vi "Get Indicators RegisterMap.vi"(8 "error in (no error)":errorcluster, 11 "Item Ref in":T1 format="%.0x") -> (0 "error out":errorcluster, 2 "Indicators RegisterMap":T2[](array[typedef]) {"Address" format="%.0x"}, 3 "Item Ref out":T1 format="%.0x")   [LabVIEW 2016, in "FPGA Addon System Explorer.lvlib"]
uses:
  FPGA Addon System Explorer.lvlib
  <vilib>/rvi/Bitfile/nirviControlStructure.ctl
  <vilib>/rvi/Bitfile/nirviTypdefDescription.ctl
  <vilib>/rvi/Bitfile/nirviMechanicalAction.ctl
  <vilib>/rvi/Bitfile/nirviSubControlStructure.ctl
  <vilib>/rvi/Bitfile/nirviClusterElementControl.ctl
  <vilib>/NI Veristand/Custom Device API/Custom Device Item Ref.ctl
  <vilib>/NI Veristand/Custom Device API/Get Item Property (Variant).vi
  Shared/Constants.vi
  Shared/FPGA Addon Shared.lvlib
  <vilib>/NI VeriStand/Custom Device API/Custom Device API.lvlib
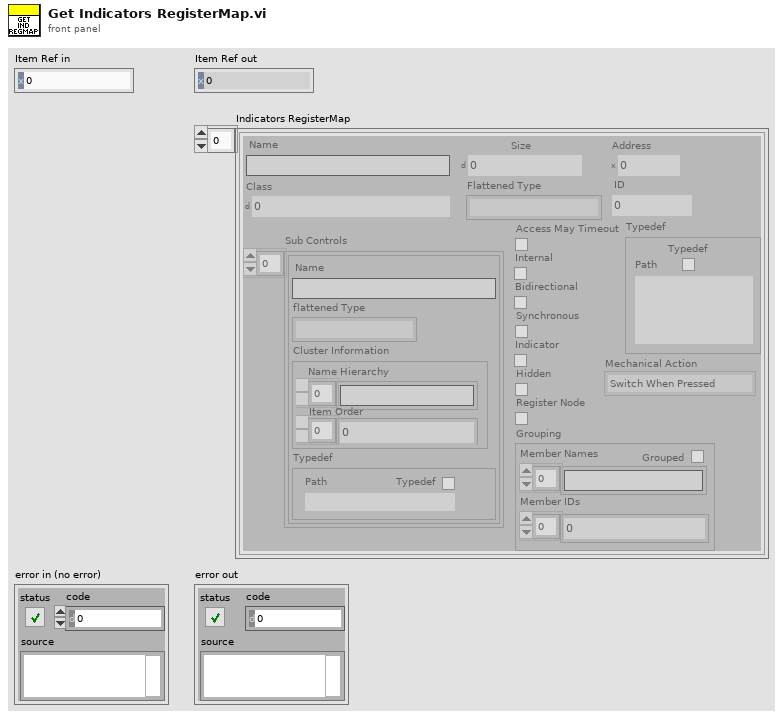
[diagram p1: front panel]
types:
  T1 = typedef "Custom Device API.lvlib/Custom Device Item Ref.ctl" = u64
  T2 = typedef "nirviControlStructure.ctl" = cluster{"Name":string, "Hidden":bool, "Indicator":bool, "Flattened Type":string, "Grouping":cluster{"Grouped":bool, "Member Names":string[], "Member IDs":u32[]}, "Address":u32, "Size":u32, "Class":u32, "Internal":bool, "Typedef":T3, "ID":u32, "Bidirectional":bool, "Synchronous":bool, "Mechanical Action":T4, "Sub Controls":T5[], "Access May Timeout":bool, "Register Node":bool}
  T3 = typedef "nirviTypdefDescription.ctl" = cluster{"Typedef":bool, "Path":path}
  T4 = typedef "nirviMechanicalAction.ctl" = enum8{"Switch When Pressed", "Switch When Released", "Switch Until Released", "Latch When Pressed", "Latch When Released", "Latch Until Released"}
  T5 = typedef "nirviSubControlStructure.ctl" = cluster{"Name":string, "flattened Type":string, "Cluster Information":T6, "Typedef":T3}
  T6 = typedef "nirviClusterElementControl.ctl" = cluster{"Name Hierarchy":string[], "Item Order":u32[]}
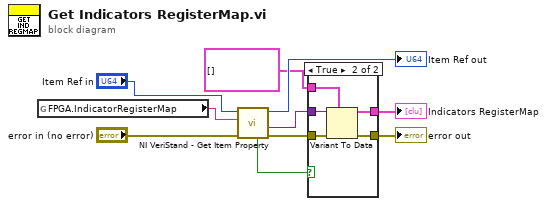
[diagram p0: block diagram]
diagram:
  n1 = global read "Constants.vi" "FPGA.IndicatorRegisterMap"() -> (w9:string)
  n2 = call-poly <vilib>:"NI VeriStand - Get Item Property.vi"("error in (no error)"="error in (no error)", "Property Name"=w9, "Item Ref in"="Item Ref in") -> ("error out"=w5:errorcluster, "Value"=w6:variant, "Item Ref out"=→"Item Ref out":T1, "Found?"=w3:bool)  [unwired: 5 in]
  n3 = case shown="True" w3 {
    tunnel: [w12 w17] -> w1
    tunnel: w6 -> [_ w16]
    tunnel: w5 -> [w11 w15]
    tunnel: [w11 w14] -> w4
    tunnel: T2[] [] ("Indicators RegisterMap") -> [w12 w13]
    frame False {
    }
    frame True {
      n4 = Variant To Data(error in=w15, type=w13, Variant=w16) -> (data=w17:T2[], error out=w14:errorcluster)
    }
  }
  "error out" <- w4
  "Indicators RegisterMap" <- w1
